vi "myRIO v1.0 Wait for RDY.vi"(8 "error in (no error)":errorcluster, 10 "timeout (ms)":i32, 11 "Generic FPGA Reference in":T1) -> (0 "error out":errorcluster, 3 "Generic FPGA Reference out":T1)   [LabVIEW 2021]
uses:
  <vilib>/myRIO/Common/Instrument Driver Framework/Utilities/typedefs/Generic FPGA Reference.ctl
  <vilib>/myRIO/Common/Instrument Driver Framework/myRIO v1.0/System/typedefs/System FPGA Reference.ctl
  <vilib>/rvi/errors/niLvFpgaAdjustHostInterfaceError.vi
  <vilib>/rvi/interface/nirviReadWriteControl/nirviReadWriteControl.xnode
  NiFpgaLv.dll
  <vilib>/rvi/interface/Simulation/niFpgaSimulationCallBeginRW.vi
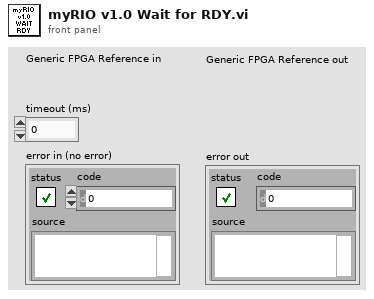
[diagram p1: front panel]
types:
  T1 = typedef "Generic FPGA Reference.ctl" = refnum<k20>
  T2 = typedef "System FPGA Reference.ctl" = refnum<k20>
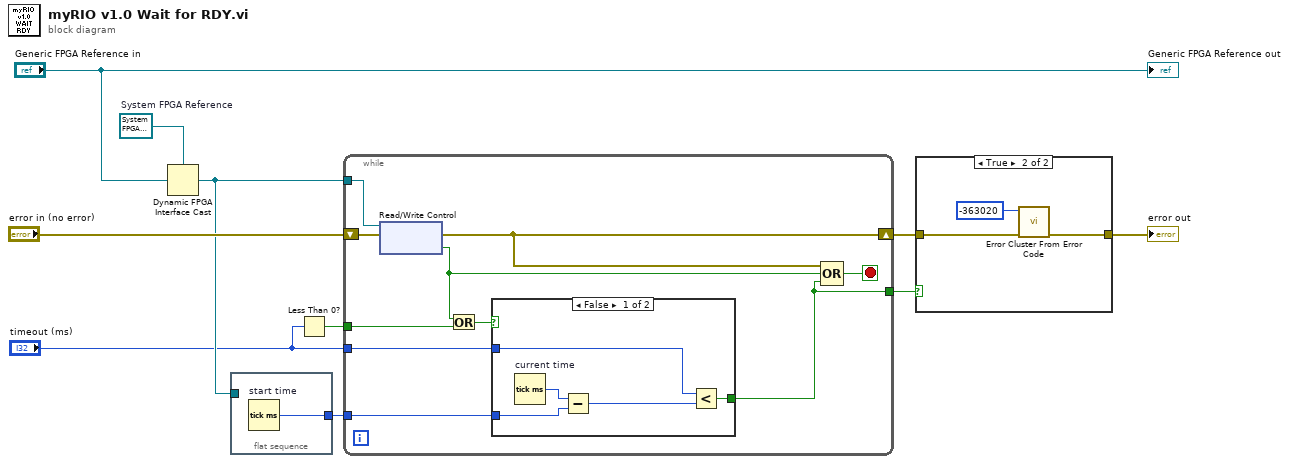
[diagram p0: block diagram]
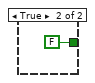
[diagram p3: hidden frame]
diagram:
  w7 = T2 refnum  # System FPGA Reference
  n1 = Dynamic FPGA Interface Cast(Session In=w7, Type="Generic FPGA Reference in") -> (Session Out=w8:T2)
  n2 = flat-sequence {
    tunnel: [w11] -> w9
    tunnel: w8 -> [_]
    frame #0 {
      n3 = Tick Count (ms) "start time"() -> (millisecond timer value=w11:u32)
    }
  }
  n4 = Less Than 0?(x="timeout (ms)") -> (x < 0?=w2:bool)
  n5 = while {
    tunnel: w8 -> [w20]
    tunnel: w9 -> [w19]
    tunnel: "timeout (ms)" -> [w18]
    tunnel: w2 -> [w16]
    shift-right: [w15] -> w4
    shift-left: "error in (no error)" -> [w21]
    tunnel: [w13] -> w1
    stop <- w14 stop-if-true
    n6 = xnode "Read/Write Control"("FPGA VI Reference In"=w20, "error in"=w21) -> ("error out"=w15:errorcluster, "SYS.RDY"=w12:bool)  [unwired: 1 out]
    n7 = Or(x=w12, y=w16) -> (x .or. y?=w17:bool)
    n8 = case shown="False" w17 {
      tunnel: w19 -> [w25 _]
      tunnel: w18 -> [w23 _]
      tunnel: [w22 FALSE] -> w13
      frame False {
        n9 = Tick Count (ms) "current time"() -> (millisecond timer value=w26:u32)
        n10 = Subtract(x=w26, y=w25) -> (x-y=w24:u32)
        n11 = Less?(x=w23, y=w24) -> (x < y?=w22:bool)
      }
      frame True {
      }
    }
    n12 = Compound Arithmetic op=OR(w15, w12, w13) -> (w14:bool)
  }
  n13 = case shown="True" w1 {
    tunnel: [w28 w30] -> w5
    tunnel: w4 -> [w28 w31]
    frame False {
    }
    frame True {
      n14 = call <vilib>:"Error Cluster From Error Code.vi"("error in (no error)"=w31, "error code (0)"=-363020) -> ("error out"=w30:errorcluster)  [unwired: 7 in]
    }
  }
  "error out" <- w5
  "Generic FPGA Reference out" <- "Generic FPGA Reference in"
